vi "Write SGL.vi"(8 "error in":errorcluster, 9 "value in":sgl, 10 "register offset":u32, 11 "session in":u32) -> (0 "error out":errorcluster, 3 "session out":u32)   [LabVIEW 2018, in "Scalar IO Operations.lvlib"]
uses:
  Scalar IO Operations.lvlib
  NiFpga.dll
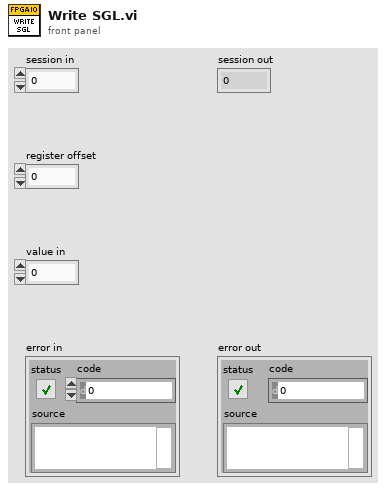
[diagram p1: front panel]
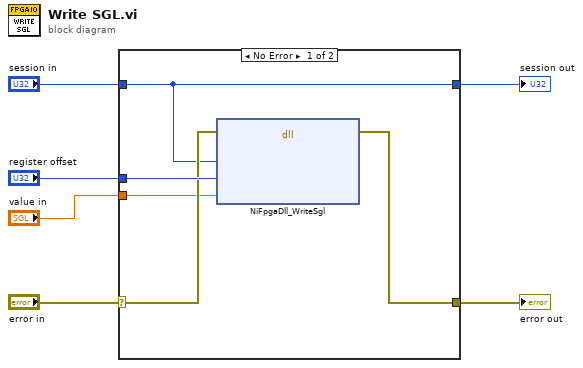
[diagram p0: block diagram]
diagram:
  n1 = case shown="No Error" "error in" {
    selector: "error in" -> [w9 w13]
    tunnel: "session in" -> [w8 w12]
    tunnel: [w11 w13] -> w5
    tunnel: "register offset" -> [w10 _]
    tunnel: [w8 w12] -> w2
    tunnel: "value in" -> [w7 _]
    frame No Error {
      n2 = dll-call lib="NiFpga.*" fn="NiFpgaDll_WriteSgl"(error in=w9, "session"=w8, "offset"=w10, "value"=w7) -> (error out=w11:errorcluster)  [unwired: 6 in, 1 out]
    }
    frame Error {
    }
  }
  "error out" <- w5
  "session out" <- w2
